vi "Custom Error Handler.vi"(8 "error in":errorcluster) -> (0 "error out":errorcluster)   [LabVIEW 2018]
doc: "Displays custom error messages for errors expected to occur during normal operation of the LabVIEW Real-Time Sequencer."
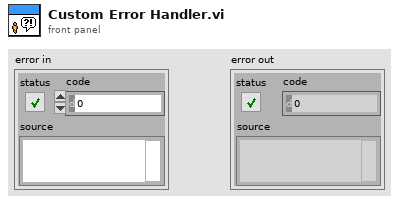
[diagram p1: front panel]
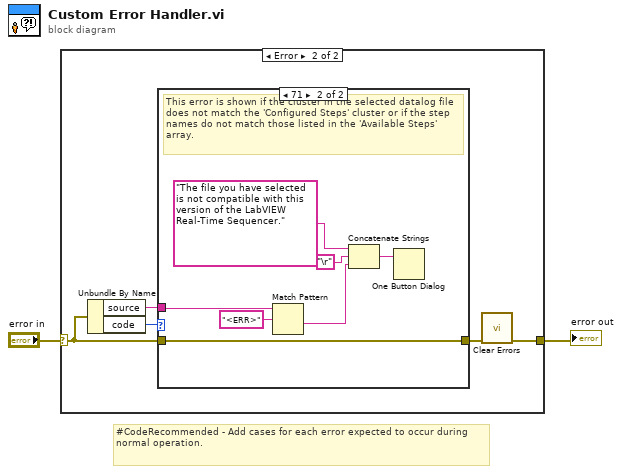
[diagram p0: block diagram]
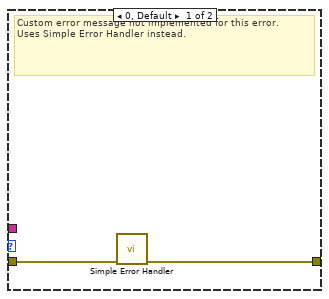
[diagram p3: hidden frame]
diagram:
  # "#CodeRecommended - Add cases for each error expected to occur during normal operation."
  n1 = case shown="Error" "error in" {
    selector: "error in" -> [w3 w6]
    tunnel: [w3 w5] -> w1
    frame No Error {
    }
    frame Error {
      n2 = Unbundle By Name(w6) -> ("source"=w4:string, "code"=w8:i32)
      n3 = case shown="71" w8 {
        tunnel: [w9 w17] -> w7
        tunnel: w6 -> [w10 w17]
        tunnel: w4 -> [_ w13]
        frame 0, Default {
          # "Custom error message not implemented for this error.\nUses Simple Error Handler instead."
          n4 = call <vilib>:"Simple Error Handler.vi"("error in (no error)"=w10) -> ("error out"=w9:errorcluster)  [unwired: 4 in, 4 out]
        }
        frame 71 {
          # "This error is shown if the cluster in the selected datalog file does not match the 'Configured Steps' cluster or if the step names do not match those listed in the 'Available Steps' array."
          n5 = Match Pattern(string=w13, regular expression="<ERR>") -> (after substring=w11:string)  [unwired: 1 in, 3 out]
          n6 = Concatenate Strings("The file you have selected is not compatible with this version of the LabVIEW Real-Time Sequencer." ("message"), "\r", w11) -> (w16:string)
          n7 = One Button Dialog(message=w16) -> ()  [unwired: 1 in, 1 out]
        }
      }
      n8 = call <vilib>:"Clear Errors.vi"("error in (no error)"=w7) -> ("error out"=w5:errorcluster)  [unwired: 5 in, 1 out]
    }
  }
  "error out" <- w1
